vi "RT Read and Parse MIDI.vi"(8 "error in":errorcluster, 11 "FPGA VI Reference In":T1) -> (0 "error out":errorcluster)   [LabVIEW 2014]
uses:
  MIDI driver/MID Command.ctl
  Controls/FPGA Reference.ctl
  <vilib>/rvi/interface/common/niFpgaWaitOnOcc.vi
  <vilib>/Utility/error.llb/Error Cluster From Error Code.vi
  <vilib>/rvi/errors/niLvFpgaAdjustHostInterfaceError.vi
  <vilib>/FPGAPlugInAG/Dynamic/niLvFpga_Close_Dynamic.vi
  <vilib>/rvi/interface/nirviMethod/nirviMethod.xnode
  <vilib>/rvi/interface/nirviCloseFPGA/nirviCloseFPGA.xnode
  <vilib>/FPGAPlugInAG/Dynamic/niLvFpga_ReadFifo_Dynamic.vi
  <vilib>/rvi/errors/niLvFpgaMergeErrorWithErrorCode.vi
  <vilib>/FPGAPlugInAG/Dynamic/niLvFpga_ConfigureFifo_Dynamic.vi
  <vilib>/FPGAPlugInAG/Dynamic/niLvFpga_StartFifo_Dynamic.vi
panel:
  out "output cluster":T2={"Device"=enum."Pads", "Parameter 1"=0, "Parameter 2"=0}
  in  "stop":bool
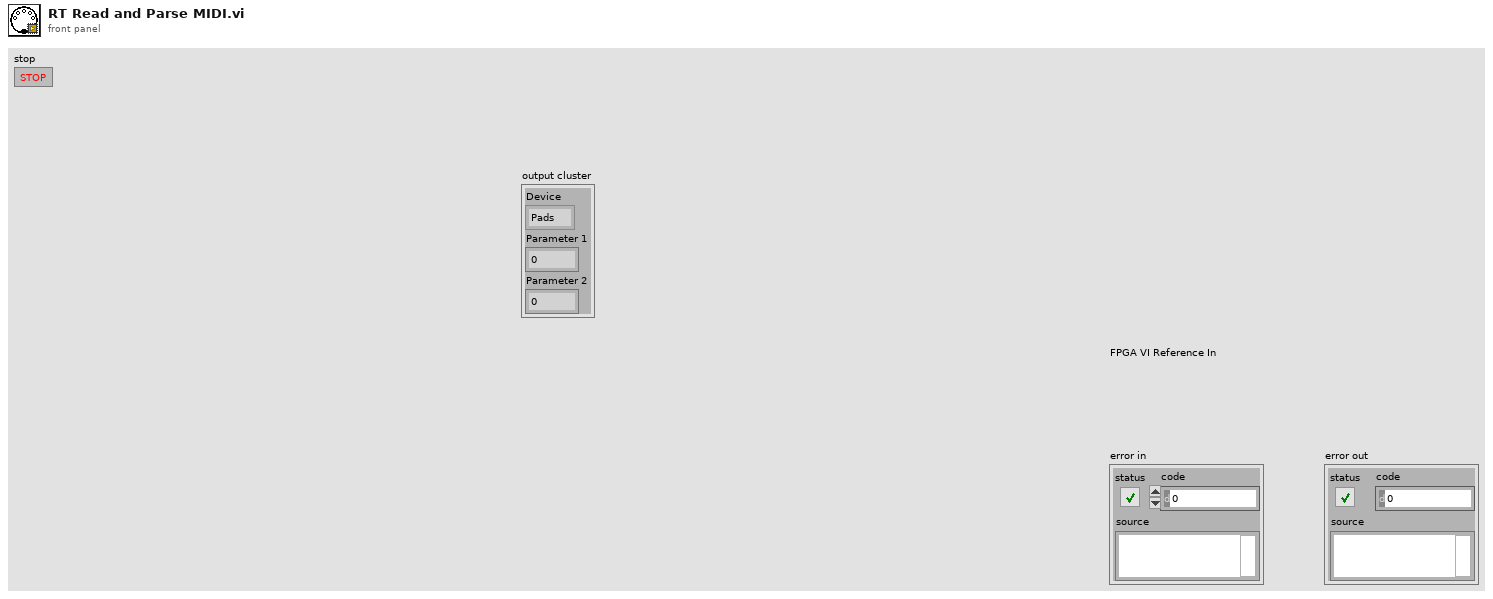
[diagram p1: front panel]
types:
  T1 = typedef "FPGA Reference.ctl" = refnum<k20>
  T2 = typedef "MID Command.ctl" = cluster{"Device":enum16{"Keys", "Controls", "Pads"}, "Parameter 1":u8, "Parameter 2":u8}
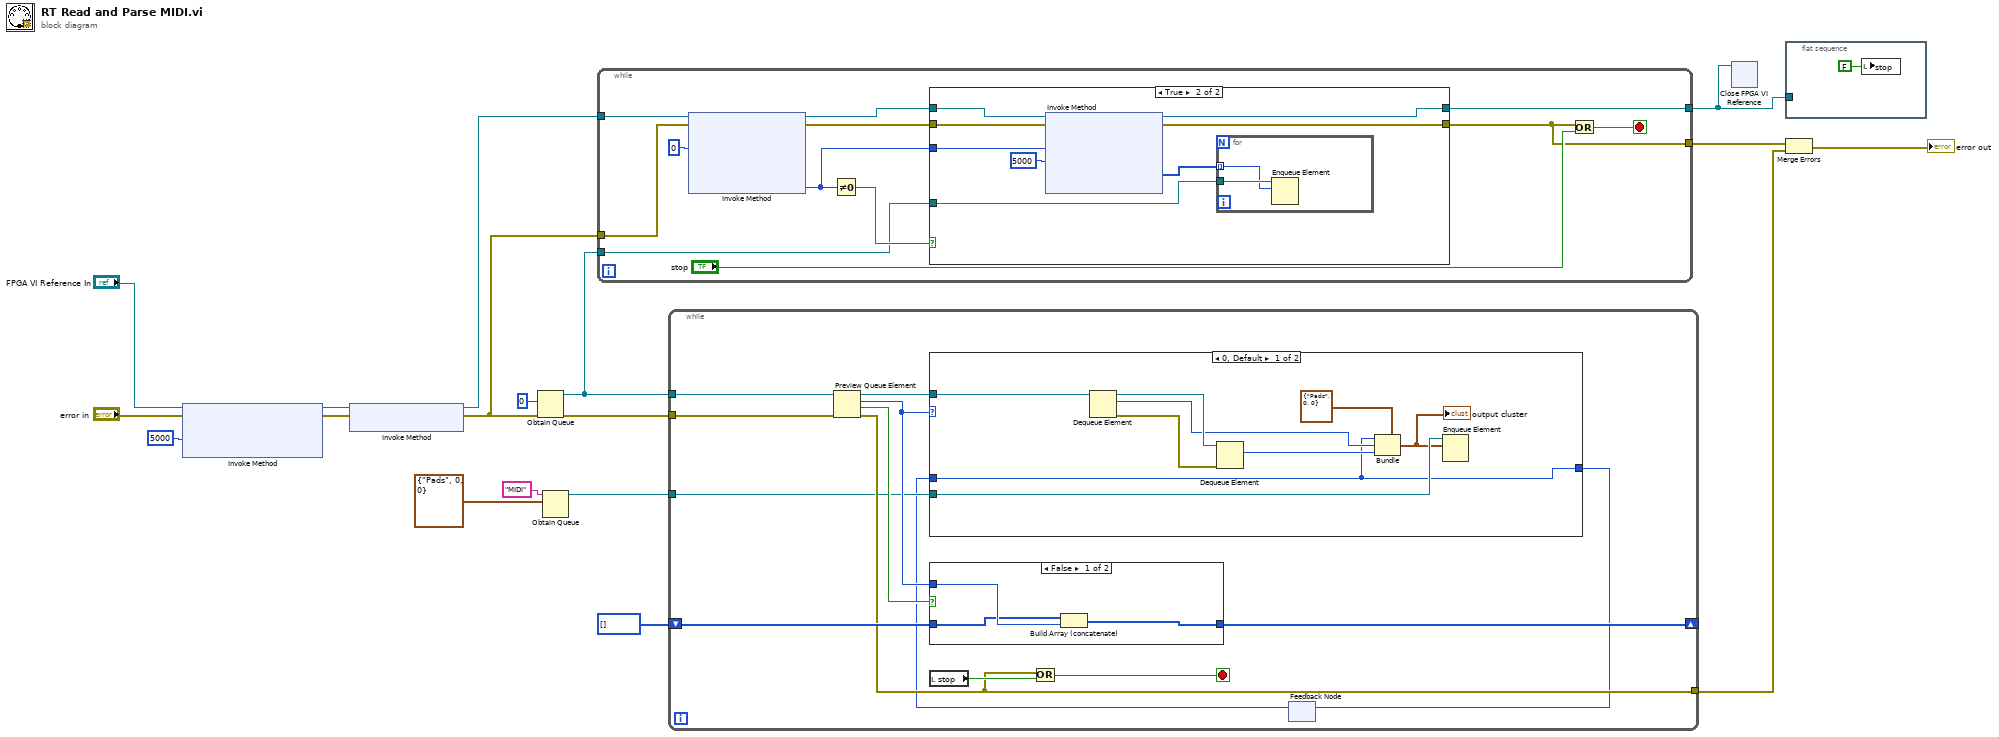
[diagram p0: block diagram]
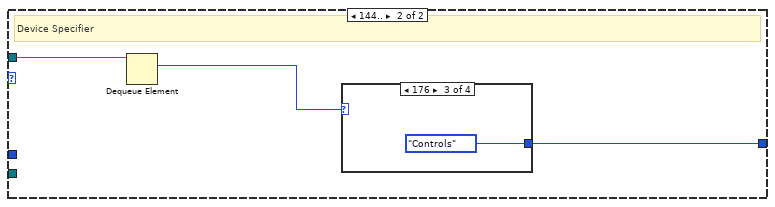
[diagram p2: hidden frame]
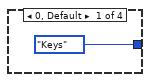
[diagram p3: hidden frame]
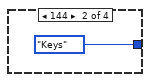
[diagram p4: hidden frame]
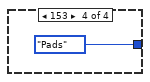
[diagram p5: hidden frame]
diagram:
  n1 = xnode "Invoke Method"("FPGA VI Reference In"="FPGA VI Reference In", "error in"="error in", "Requested Depth"=u32 5000) -> ("FPGA VI Reference Out"=w18:T1, "error out"=w12:errorcluster)  [unwired: 1 out]
  n2 = xnode "Invoke Method"("FPGA VI Reference In"=w18, "error in"=w12) -> ("FPGA VI Reference Out"=w17:T1, "error out"=w11:errorcluster)
  n3 = Obtain Queue(element data type=u8 0, error in (no error)=w11) -> (queue out=w14:refnum<queue>, error out=w10:errorcluster)  [unwired: 3 in, 1 out]
  n4 = Obtain Queue(name (unnamed)="MIDI", element data type=T2 {"Device"=enum."Pads", "Parameter 1"=0, "Parameter 2"=0} ("MIDI Command")) -> (queue out=w5:refnum<queue>)  [unwired: 3 in, 2 out]
  n5 = while {
    tunnel: w17 -> [w30]
    tunnel: [w26] -> w13
    tunnel: w14 -> [w24]
    tunnel: w11 -> [w23]
    tunnel: [w19] -> w9
    stop <- w20 stop-if-true
    n6 = xnode "Invoke Method"("FPGA VI Reference In"=w30, "error in"=w23, "Number of Elements"=u32 0) -> ("FPGA VI Reference Out"=w27:T1, "error out"=w22:errorcluster, "Elements Remaining"=w25:u32)  [unwired: 1 in, 1 out]
    n7 = Not Equal To 0?(x=w25) -> (x != 0?=w28:bool)
    n8 = case shown="True" w28 {
      tunnel: w27 -> [w32 w40]
      tunnel: [w32 w39] -> w26
      tunnel: w25 -> [_ w38]
      tunnel: w24 -> [_ w36]
      tunnel: w22 -> [w31 w34]
      tunnel: [w31 w33] -> w19
      frame False {
      }
      frame True {
        n9 = xnode "Invoke Method"("FPGA VI Reference In"=w40, "error in"=w34, "Number of Elements"=w38, "Timeout (ms)"=5000) -> ("FPGA VI Reference Out"=w39:T1, "error out"=w33:errorcluster, "Data"=w35:u8[])  [unwired: 1 out]
        n10 = for {
          tunnel: w36 -> [w42]
          tunnel: w35 -> [w41] mode=indexing
          n11 = Enqueue Element(queue=w42, element=w41) -> ()  [unwired: 2 in, 3 out]
        }
      }
    }
    n12 = Or(x=w19, y="stop") -> (x .or. y?=w20:bool)
  }
  n13 = while {
    tunnel: w14 -> [w55]
    tunnel: w10 -> [w54]
    shift-right: [w50] -> _
    shift-left: u8[] [] ("appended array") -> [w51]
    tunnel: [w49] -> w6
    tunnel: w5 -> [w45]
    stop <- w52 stop-if-true
    n14 = Preview Queue Element(queue=w55, error in (no error)=w54) -> (queue out=w47:refnum<queue>, element=w46:u8, timed out?=w48:bool, error out=w49:errorcluster)  [unwired: 1 in]
    n15 = case shown="False" w48 {
      tunnel: w46 -> [w74 _]
      tunnel: w51 -> [w73 w75]
      tunnel: [w72 w75] -> w50
      frame False {
        n16 = Build Array (concatenate)(w73, w74) -> (w72:u8[])
      }
      frame True {
      }
    }
    n17 = local read "stop"() -> (w53:bool)
    n18 = Or(x=w49, y=w53) -> (x .or. y?=w52:bool)
    n19 = feedback #1() -> (w43:enum16{"Keys", "Controls", "Pads"})  [unwired: 1 in]
    n20 = case shown="0, Default" w46 {
      tunnel: w47 -> [w64 w67]
      tunnel: w45 -> [w60 _]
      tunnel: [w56 w65] -> w44
      tunnel: w43 -> [w56 _]
      frame 0, Default {
        n21 = Dequeue Element(queue=w64) -> (queue out=w63:refnum<queue>, element=w57:u8, error out=w62:errorcluster)  [unwired: 2 in, 1 out]
        n22 = Dequeue Element(queue=w63, error in (no error)=w62) -> (element=w58:u8)  [unwired: 1 in, 3 out]
        n23 = Bundle(cluster=T2 {"Device"=enum."Pads", "Parameter 1"=0, "Parameter 2"=0} ("MIDI Command"), "Device"=w56, "Parameter 1"=w57, "Parameter 2"=w58) -> (w59:T2)
        "output cluster" <- w59
        n24 = Enqueue Element(queue=w60, element=w59) -> ()  [unwired: 2 in, 3 out]
      }
      frame 144.. {
        # "Device Specifier"
        n25 = Dequeue Element(queue=w67) -> (element=w66:u8)  [unwired: 2 in, 3 out]
        n26 = case shown="176" w66 {
          tunnel: [enum16{"Keys", "Controls", "Pads"}."Keys" enum16{"Keys", "Controls", "Pads"}."Keys" enum16{"Keys", "Controls", "Pads"}."Controls" enum16{"Keys", "Controls", "Pads"}."Pads"] -> w65
          frame 0, Default {
          }
          frame 144 {
          }
          frame 176 {
          }
          frame 153 {
          }
        }
      }
    }
    n27 = feedback-in #1(w44) -> ()
  }
  n28 = xnode "Close FPGA VI Reference"("FPGA VI Reference In"=w13) -> ()  [unwired: 1 in, 1 out]
  n29 = flat-sequence {
    tunnel: w13 -> [_]
    frame #0 {
      n30 = local write "stop"(FALSE ("stop")) -> ()
    }
  }
  n31 = Merge Errors(w9, w6) -> (→"error out":errorcluster)
